vi "Table, Copy Row Values.vi"(5 "n rows (1)":i32=1, 6 "error in":errorcluster, 7 "row (0)":i32, 8 "Tbl Refnum Dst":refnum<vi>, 9 "Tbl Refnum Src":refnum<vi>) -> (0 "error out":errorcluster, 2 "Tbl Refnum Dst out":refnum<vi>, 3 "Tbl Refnum Src out":refnum<vi>)   [LabVIEW 2010]
doc: "This function copies one of more rows of the source table to the destination table."
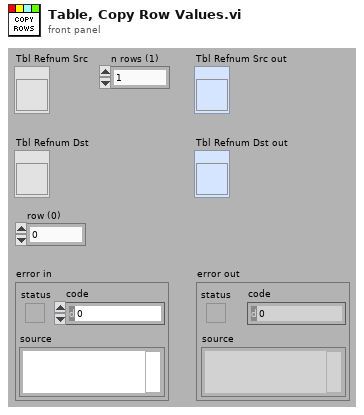
[diagram p1: front panel]
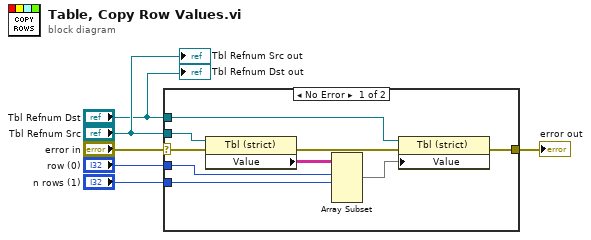
[diagram p0: block diagram]
diagram:
  n1 = case shown="No Error" "error in" {
    selector: "error in" -> [w11 w16]
    tunnel: [w14 w16] -> w6
    tunnel: "Tbl Refnum Dst" -> [w8 _]
    tunnel: "Tbl Refnum Src" -> [w9 _]
    tunnel: "n rows (1)" -> [w10 _]
    tunnel: "row (0)" -> [w7 _]
    frame No Error {
      n2 = property class="Tbl (strict)"(reference=w9, error in=w11) -> (error out=w15:errorcluster, "Value"=w13:string[][])  [unwired: 1 out]
      n3 = Array Subset "Array Subset"(array=w13, index (row)=w7, length (row)=w10) -> (w12:string[][])  [unwired: 2 in]
      n4 = property class="Tbl (strict)"(reference=w8, error in=w15, "Value"=w12) -> (error out=w14:errorcluster)  [unwired: 1 out]
    }
    frame Error {
    }
  }
  "error out" <- w6
  "Tbl Refnum Src out" <- "Tbl Refnum Src"
  "Tbl Refnum Dst out" <- "Tbl Refnum Dst"
